vi "Renishaw-XL80_SetAutoCompensationMode.vi"(8 "error in (no error)":errorcluster, 10 "AutoCompensationMode":i32(ring) items=["AUTO_COMPENSATION_OFF"=0, "AUTO_COMPENSATION_AIR"=1, "AUTO_COMPENSATION_FULL"=3], 11 "Renishaw-XL80_EMU in":refnum<class "Renishaw-XL80_EMU.lvclass">) -> (0 "error out":errorcluster, 3 "Renishaw-XL80_EMU out":refnum<class "Renishaw-XL80_EMU.lvclass">)   [LabVIEW 2024, in "Renishaw-XL80_EMU.lvclass"]
doc: "Writing this property will set the current compensation mode.\n\nDefinition\nHRESULT\nput_AutoCompensationMode(\n [in] AUTO_COMPENSATION_MODES newVal\n);\nParameters\nnewVal\nSpecifies the compensation mode to use. Must be one of the values specified by the enumerated type AUTO_COMPENSATION_MODES.\n\nComments\nThis property will return with an HRESULT of E_INVALIDARG if newVal specifies a value that is not a member of the enumerated type AUTO_COMPENSATION_MODES.\n\nThis property will return with an HRESULT of E_FAIL if the current MeasurementMode is set to MEASUREMENT_ANGULAR and newVal is set to AUTO_COMPENSATION_FULL.\n\nIf the client sets AutoCompensationMode to AUTO_COMPENSATION_FULL then both lambda and the material compensation factor will be updated immediately and then automatically as new environmental values arrive.\n\nIf the client sets AutoCompensationMode to AUTO_COMPENSATION_AIR then lambda will be updated immediately and then automatically as new environmental values arrive. The material compensation factor will no longer be updated automatically. It will remain at its last updated value.\n\nIf the client sets AutoCompensationMode to AUTO_COMPENSATION_OFF then lambda and the material compensation factor will cease to be updated automatically. They will remain at their last updated values.\n\nIf the property is successful it will return with an HESULT of S_OK."
uses:
  Renishaw-XL80_EMU.lvclass
  Renishaw-XL80_EMU.lvclass/Renishaw-XL80_EMU.ctl
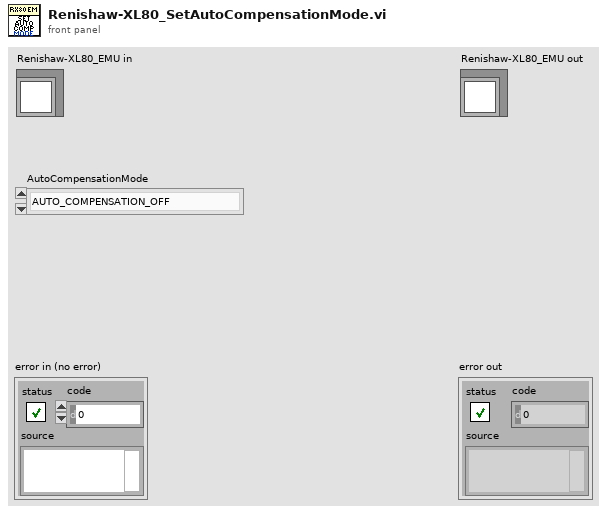
[diagram p1: front panel]
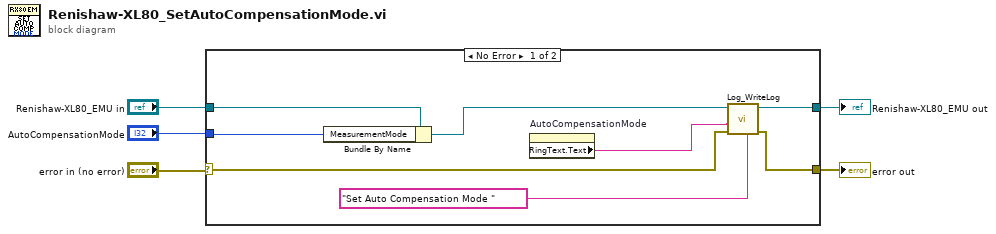
[diagram p0: block diagram]
diagram:
  n1 = case shown="No Error" "error in (no error)" {
    selector: "error in (no error)" -> [w10 w14]
    tunnel: [w11 w15] -> w5
    tunnel: "Renishaw-XL80_EMU in" -> [w13 w15]
    tunnel: [w9 w14] -> w2
    tunnel: "AutoCompensationMode" -> [w8 _]
    frame No Error {
      n2 = Bundle By Name(cluster=w13, "MeasurementMode"=w8) -> (w12:refnum<class "Renishaw-XL80_EMU.lvclass">)
      n3 = property on="AutoCompensationMode" class="Ring (strict)"() -> ("RingText.Text"=w6:string)  [unwired: 2 in, 2 out]
      n4 = call-dynamic "Log_WriteLog.vi"("Additional text"="Set Auto Compensation Mode ", "error in (no error)"=w10, "Response"=w6, "Log in"=w12) -> ("error out"=w9:errorcluster, "Log out"=w11:refnum<class "Renishaw-XL80_EMU.lvclass">)  [unwired: 6 in]
    }
    frame Error {
    }
  }
  "error out" <- w2
  "Renishaw-XL80_EMU out" <- w5
